vi "Log Warning.vi"(7 "Source":string, 8 "error in (no error)":errorcluster, 10 "Message":string, 11 "Logging In":refnum<class "Logging.lvclass">) -> (0 "error out":errorcluster, 3 "Logging Out":refnum<class "Logging.lvclass">)   [LabVIEW 2021, in "Logging.lvclass"]
doc: "Enter a warning-level message into the system log.\nA warning is an indication that something unexpected happened, or indicative of some problem in the near future (e.g. ‘disk space low’). The software is still working as expected."
uses:
  Logging.lvclass
  Protected/Level.ctl
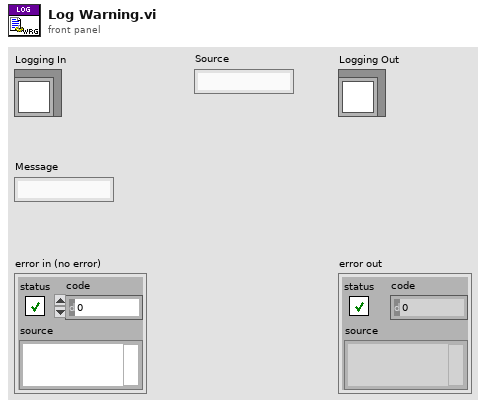
[diagram p1: front panel]
types:
  T1 = typedef "Logging.lvclass/Level.ctl" = enum16{"DEBUG", "INFO", "WARNING", "ERROR", "CRITICAL"}
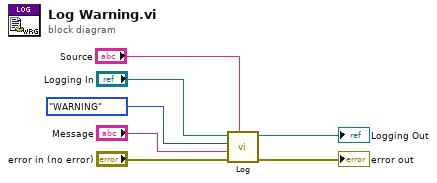
[diagram p0: block diagram]
diagram:
  n1 = call-dynamic "Log.vi"("Source"="Source", "error in (no error)"="error in (no error)", "Message"="Message", "Level"=Level."WARNING", "Logging In"="Logging In") -> ("error out"=→"error out":errorcluster, "Logging Out"=→"Logging Out":refnum<class "Logging.lvclass">)  [unwired: 5 in]
